vi "Char to Modbus.vi"(10 "Unsigned Char":string) -> (2 "Char Register Out":u16 format="%016b")   [LabVIEW 2024, in "Bronkhorst Flexi-Flow ModbusTCP API.lvlib"]
uses:
  Bronkhorst Flexi-Flow ModbusTCP API.lvlib
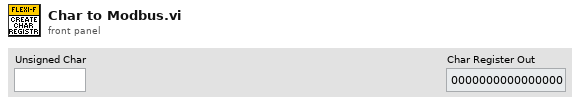
[diagram p1: front panel]
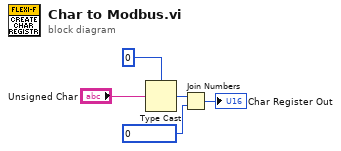
[diagram p0: block diagram]
diagram:
  n1 = Type Cast(type=u8 0, x="Unsigned Char") -> (*(type *) &x=w2:u8)
  n2 = Join Numbers(hi=w2, lo=u8 0 ("hi")) -> ((hi.lo)=→"Char Register Out":u16)
